vi "oa_Get DSA 9229 Oversample Rate and Filter Delay.vi"(11 "set sample rate":dbl) -> (0 "input delay":dbl, 1 "SampClkTimebase":dbl, 2 "Actual Sample Rate":dbl, 3 "oversample rate":dbl)   [LabVIEW 2017, in "SoundVib_TachProcess.lvlib"]
uses:
  <vilib>/addons/Sound and Vibration/Order Analysis/Tach Process/SoundVib_TachProcess.lvlib
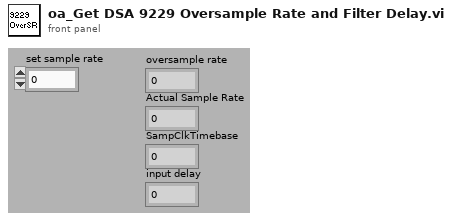
[diagram p1: front panel]
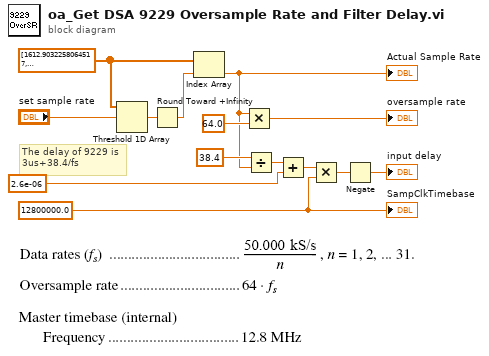
[diagram p0: block diagram]
diagram:
  w8 = dbl[] [1612.9032258064517, 1666.6666666666667, 1724.1379310344828, 1785.7142857142858, 1851.851851851852, 1923.076923076923, 2000.0, 2083.3333333333335, 2173.913043478261, 2272.7272727272725, 2380.9523809523807, 2500.0, 2631.5789473684213, 2777.777777777778, 2941.176470588235, 3125.0, 3333.3333333333335, 3571.4285714285716, 3846.153846153846, 4166.666666666667, 4545.454545454545, 5000.0, 5555.555555555556, 6250.0, 7142.857142857143, 8333.333333333334, 10000.0, 12500.0, 16666.666666666668, 25000.0, 50000.0] ("reversed array")
  w1 = 12800000.0 ("y")
  # "The delay of 9229 is\n3us+38.4/fs"
  n1 = Threshold 1D Array(2:"set sample rate", 3:w8) -> (0:w14:dbl)  [unwired: 1 in]
  n2 = Round Toward +Infinity(x=w14) -> (ceil(x): smallest int >= x=w13:dbl)
  n3 = Index Array(array=w8, index=w13) -> (element=w4:dbl)
  "Actual Sample Rate" <- w4
  n4 = Multiply(x=w4, y=64.0) -> (x*y=→"oversample rate":dbl)
  n5 = Divide(x=38.4 ("y"), y=w4) -> (x/y=w3:dbl)
  n6 = Add(x=w3, y=2.6e-06) -> (x+y=w6:dbl)
  n7 = Multiply(x=w6, y=w1) -> (x*y=w2:dbl)
  n8 = Negate(x=w2) -> (-x=→"input delay":dbl)
  "SampClkTimebase" <- w1
